vi "Enable Live Comm.vi"(8 "error in":errorcluster, 11 "TEC 1090 in":refnum<class "Meerstetter TEC.lvclass">) -> (0 "error out":errorcluster, 3 "TEC 1090 out":refnum<class "Meerstetter TEC.lvclass">)   [LabVIEW 2014, in "Meerstetter Lib.lvlib" / "Meerstetter TEC.lvclass"]
uses:
  Meerstetter TEC.lvclass
  reusable/Session APIs/Serial/Serial Session.lvclass
  Configurable Device/Configurable Device.lvclass/Configurable Device.ctl
  Meerstetter TEC.lvclass/Meerstetter TEC.ctl
  Configurable Device/Read Log Session.vi
  Accessors/Read SerialSession.vi
  reusable/Session APIs/Serial/Public/Asynchronous Write.vi
  reusable/Session APIs/Serial/Public/Asynchronous Read.vi
  <userlib>/_Session Fwk/Session - Root.lvclass
  reusable/Session APIs/Session Log/System Log.lvclass
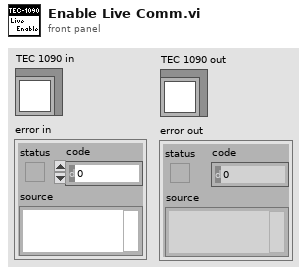
[diagram p1: front panel]
types:
  T1 = typedef "Session - Root.lvclass/Session Handle.ctl" = refnum<data-value>
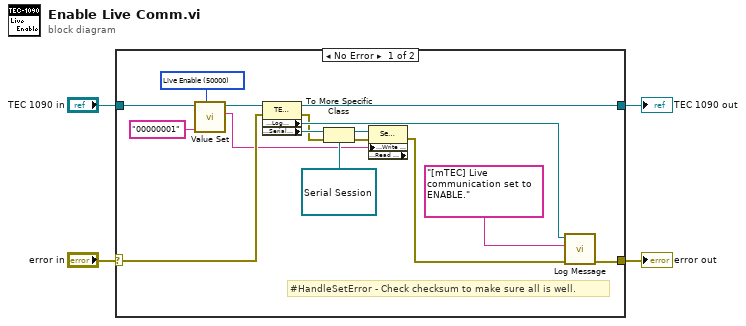
[diagram p0: block diagram]
diagram:
  n1 = case shown="No Error" "error in" {
    selector: "error in" -> [w17 w22]
    tunnel: [w11 w22] -> w3
    tunnel: [w13 w21] -> w1
    tunnel: "TEC 1090 in" -> [w20 w21]
    frame No Error {
      w19 = u16 50000 items=["Input Selection"=2000, "Status"=2010, "Set Current"=2020, "Set Voltage"=2021, "Current Limitation"=2030, "Voltage Limitation"=2031, "Current Error Threshold"=2032, "Voltage Error Threshold"=2033, "Channel Baud Rate"=2050, "Response Delay"=2052, "Timeout"=2060, "Target Object Temperature"=3000, "Coarse Temp Ramp"=3003, "Proximity Width"=3002, "Kp"=3010, "Ti"=3011, "Td"=3012, "D Part Damping D1"=3013, "Live Enable"=50000, "Live Set Current"=50001, "Live Set Voltage"=50002, "Object Target Temperature"=50012, "Save Data to Flash"=108] ("Value Set")
      # "#HandleSetError - Check checksum to make sure all is well."
      n2 = call "Value Set.vi"("Value Set"=w19, "Value"="00000001", "TEC 1090"=w20) -> ("hex integer string"=w12:string, "TEC 1091"=w18:refnum<class "Meerstetter TEC.lvclass">)  [unwired: 7 in]
      n3 = property class="TEC 1090"(reference=w18, error in=w17) -> (reference out=w13:refnum<class "Meerstetter TEC.lvclass">, error out=w5:errorcluster, "Accessors:Log Session"=w6:T1, "Accessors:SerialSession"=w7:T1)
      n4 = To More Specific Class(target class=refnum<data-value> refnum, reference=w7, error in=w5) -> (specific class reference=w15:refnum<data-value>, error out=w14:errorcluster)
      n5 = property class="Serial Session" props=["Public:Write - Asynchronous", "Public:Read - Asynchronous"](reference=w15, error in=w14, "Public:Write - Asynchronous"=w12) -> (error out=w9:errorcluster)  [unwired: 2 out]
      n6 = call "Log Message.vi"("error in"=w9, "MSG In"="[mTEC] Live communication set to ENABLE." ("format string"), "session in"=w6) -> ("error out"=w11:errorcluster)  [unwired: 7 in, 1 out]
    }
    frame Error {
    }
  }
  "error out" <- w3
  "TEC 1090 out" <- w1
